vi "test Initialize and Finalize Hardware_Invalid Module.vi"(8 "error in":errorcluster, 11 "test case in":refnum<class "Hardware API.lvclass">) -> (0 "error out":errorcluster, 3 "test case out":refnum<class "Hardware API.lvclass">)   [LabVIEW 2020, in "Hardware API.lvclass"]
uses:
  Hardware API.lvclass
  <vilib>/addons/_JKI Toolkits/VI Tester/TestCase.llb/TestCase.lvclass
  Hardware API/AIM ARINC 429 Hardware API.lvlib
  C:/Program Files (x86)/National Instruments/LabVIEW 2020/vi.lib/addons/_JKI Toolkits/VI Tester/TestCase.llb/TestCase.lvclass
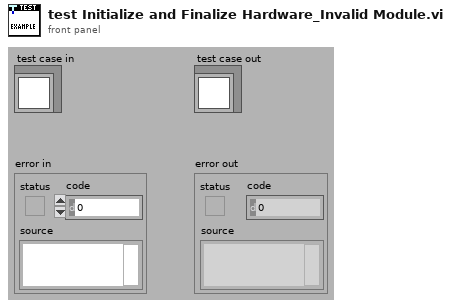
[diagram p1: front panel]
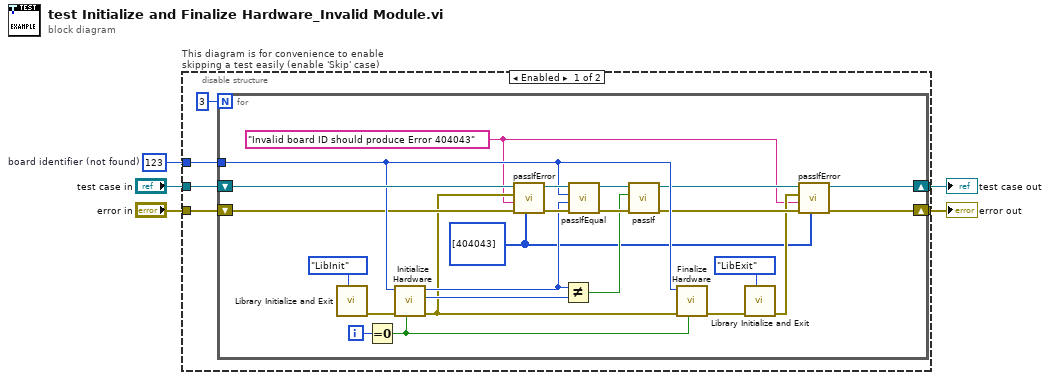
[diagram p0: block diagram]
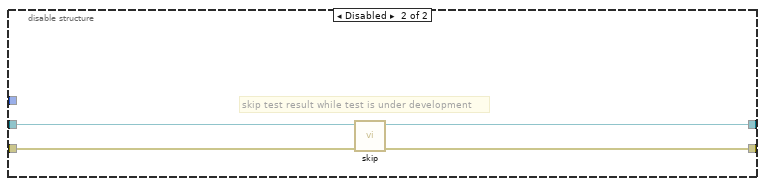
[diagram p2: hidden frame]
diagram:
  w1 = u8 123  # board identifier (not found)
  n1 = disable-structure "This diagram is for convenience to enable skipping a test easily (enable 'Skip' case)" shown="Enabled" {
    disable-tunnel: "test case in" -> [w11 w39]
    disable-tunnel: [w8 w37] -> w2
    disable-tunnel: [w9 w38] -> w4
    disable-tunnel: "error in" -> [w10 w36]
    disable-tunnel: w1 -> [w7 _]
    frame Enabled {
      n2 = for {
        N: 3 -> [_]
        tunnel: w7 -> [w28]
        shift-right: [w17] -> w8
        shift-left: w11 -> [w35]
        shift-right: [w18] -> w9
        shift-left: w10 -> [w22]
        i -> [w13]
        w15 = "Invalid board ID should produce Error 404043" ("task (\"\")")
        w14 = i32[] [404043] ("passing error codes (default = any error code)")
        n3 = call "Library Initialize and Exit.vi"("action"=enum16{"LibInit", "LibExit"}."LibInit") -> ("error out"=w24:errorcluster)  [unwired: 8 in, 2 out]
        n4 = Equal To 0?(x=w13) -> (x = 0?=w12:bool)
        n5 = call "Initialize Hardware.vi"("reset (F)"=w12, "error in"=w24, "board identifier in"=w28) -> ("error out"=w20:errorcluster, "module handle out"=w26:u8, "board identifier out"=w27:u8)  [unwired: 6 in]
        n6 = call-dynamic "passIfError.vi"("passing error codes (default = any error code)"=w14, "error in (no error)"=w22, "task (\"\")"=w15, "error"=w20, "TestCase in"=w35) -> ("error out"=w30:errorcluster, "TestCase out"=w29:refnum<class "Hardware API.lvclass">)  [unwired: 5 in]
        n7 = Not Equal?(x=w27, y=w26) -> (x != y?=w25:bool)
        n8 = call-dynamic "passIfEqual.vi"("error in (no error)"=w30, "y"=w27, "x"=w28, "TestCase in"=w29) -> ("error out"=w32:errorcluster, "TestCase out"=w31:refnum<class "Hardware API.lvclass">)  [unwired: 6 in]
        n9 = call-dynamic "passIf.vi"("error in (no error)"=w32, "pass"=w25, "TestCase in"=w31) -> ("error out"=w23:errorcluster, "TestCase out"=w21:refnum<class "Hardware API.lvclass">)  [unwired: 7 in]
        n10 = call "Finalize Hardware.vi"("force (F)"=w12, "error in"=w20, "board identifier"=w28) -> ("error out"=w19:errorcluster)  [unwired: 8 in]
        n11 = call "Library Initialize and Exit.vi"("action"=enum16{"LibInit", "LibExit"}."LibExit", "error in"=w19) -> ("error out"=w16:errorcluster)  [unwired: 7 in, 2 out]
        n12 = call-dynamic "passIfError.vi"("passing error codes (default = any error code)"=w14, "error in (no error)"=w23, "task (\"\")"=w15, "error"=w16, "TestCase in"=w21) -> ("error out"=w18:errorcluster, "TestCase out"=w17:refnum<class "Hardware API.lvclass">)  [unwired: 5 in]
      }
    }
    frame Disabled {
      # "skip test result while test is under development"
      n13 = call <vilib>:"skip.vi"("error in (no error)"=w36, "TestCase in"=w39) -> ("error out"=w38:errorcluster, "TestCase out"=w37:refnum<class "Hardware API.lvclass">)  [unwired: 8 in]
    }
  }
  "error out" <- w4
  "test case out" <- w2
